vi "dfd_ZP Add Unit Circle and Axises.vi"(8 "error in (no error)":errorcluster, 10 "upper half plane only":bool, 11 "zero pole plot in":cluster{dbl[], dbl[]}[](array[cluster])) -> (0 "error out":errorcluster, 3 "zero pole plot out":cluster{dbl[], dbl[]}[](array[cluster]))   [LabVIEW 2017, in "NI_DigFilterLicensed.lvlib"]
uses:
  <vilib>/addons/Digital Filter Design/NI_DigFilterLicensed.lvlib
  <vilib>/Analysis/NI_AALBase.lvlib
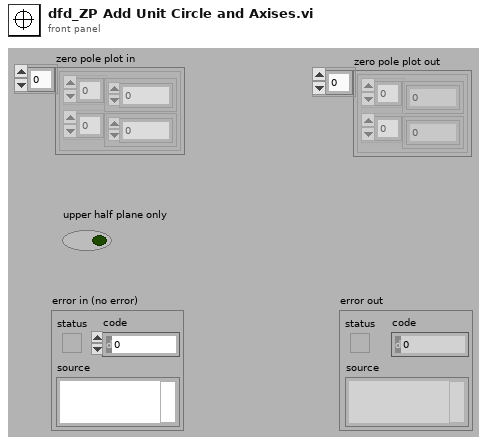
[diagram p1: front panel]
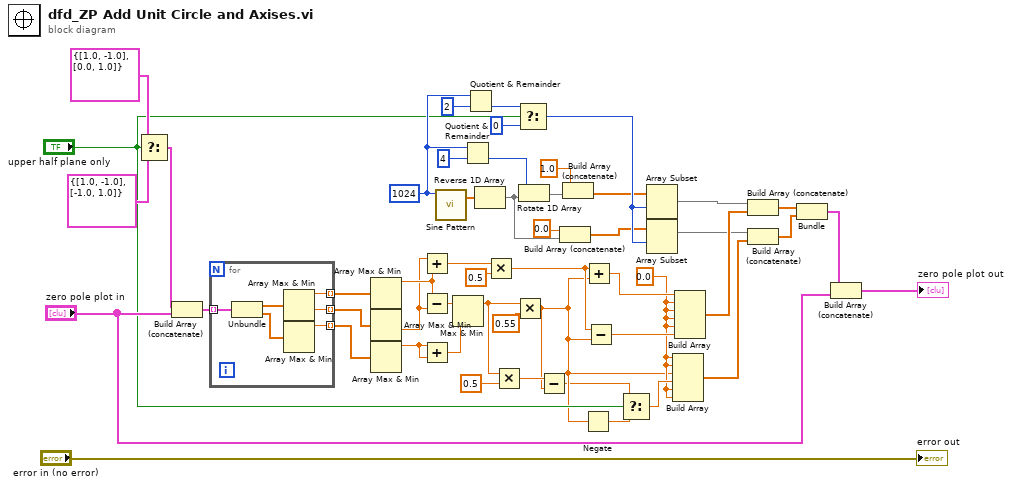
[diagram p0: block diagram]
diagram:
  w24 = 0.0 ("element")
  w22 = 1024 ("samples")
  n1 = Select(t=cluster{dbl[], dbl[]} {[1.0, -1.0], [0.0, 1.0]}, s="upper half plane only", f=cluster{dbl[], dbl[]} {[1.0, -1.0], [-1.0, 1.0]}) -> (s? t:f=w27:cluster{dbl[], dbl[]})
  n2 = Build Array (concatenate)(w27, "zero pole plot in") -> (w44:cluster{dbl[], dbl[]}[])
  n3 = for {
    tunnel: w44 -> [w57] mode=indexing
    tunnel: [w54] -> w42 mode=indexing
    tunnel: [w53] -> w41 mode=indexing
    tunnel: [w52] -> w40 mode=indexing
    n4 = Unbundle(w57) -> (w56:dbl[], w55:dbl[])
    n5 = Array Max & Min(array=w56) -> (max value=w54:dbl, min value=w53:dbl)  [unwired: 2 out]
    n6 = Array Max & Min(array=w55) -> (max value=w52:dbl)  [unwired: 3 out]
  }
  n7 = Array Max & Min(array=w42) -> (max value=w34:dbl)  [unwired: 3 out]
  n8 = Array Max & Min(array=w41) -> (min value=w33:dbl)  [unwired: 3 out]
  n9 = Array Max & Min(array=w40) -> (max value=w37:dbl)  [unwired: 3 out]
  n10 = Add(x=w33, y=w34) -> (x+y=w31:dbl)
  n11 = Subtract(x=w34, y=w33) -> (x-y=w39:dbl)
  n12 = Add(x=w37, y=w37) -> (x+y=w38:dbl)
  n13 = call <vilib>:"Sine Pattern.vi"("samples"=w22) -> ("Sinusoidal Pattern"=w10:dbl[])  [unwired: 3 in, 1 out]
  n14 = Max & Min(x=w39, y=w38) -> (max(x,y)=w19:dbl)  [unwired: 1 out]
  n15 = Quotient & Remainder(x=w22, y=4) -> (floor(x/y)=w9:i32)  [unwired: 1 out]
  n16 = Quotient & Remainder(x=w22, y=2) -> (floor(x/y)=w20:i32)  [unwired: 1 out]
  n17 = Reverse 1D Array(array=w10) -> (reversed array=w4:dbl[])
  n18 = Multiply(x=w31, y=0.5) -> (x*y=w30:dbl)
  n19 = Multiply(x=w19, y=0.5) -> (x*y=w17:dbl)
  n20 = Multiply(x=w19, y=0.55) -> (x*y=w16:dbl)
  n21 = Select(t=w20, s="upper half plane only", f=0) -> (s? t:f=w13:i32)
  n22 = Rotate 1D Array(1:w4, 2:w9) -> (0:w6:dbl[])
  n23 = Subtract(x=w17, y=w16) -> (x-y=w15:dbl)
  n24 = Build Array (concatenate)(0.0, w4) -> (w7:dbl[])
  n25 = Build Array (concatenate)(1.0, w6) -> (w5:dbl[])
  n26 = Negate(x=w16) -> (-x=w26:dbl)
  n27 = Add(x=w30, y=w16) -> (x+y=w49:dbl)
  n28 = Subtract(x=w30, y=w16) -> (x-y=w36:dbl)
  n29 = Select(t=w15, s="upper half plane only", f=w26) -> (s? t:f=w25:dbl)
  n30 = Array Subset(array=w5, index=w13) -> (w12:dbl[])  [unwired: 1 in]
  n31 = Array Subset(array=w7, index=w13) -> (w8:dbl[])  [unwired: 1 in]
  n32 = Build Array(w24, w24, w16, w25, w24, w24) -> (w11:dbl[])
  n33 = Build Array(w49, w24, w24, w24, w24, w36) -> (w48:dbl[])
  n34 = Build Array (concatenate)(w12, w48) -> (w47:dbl[])
  n35 = Build Array (concatenate)(w8, w11) -> (w46:dbl[])
  n36 = Bundle(w47, w46) -> (w1:cluster{dbl[], dbl[]})  [unwired: 1 out]
  n37 = Build Array (concatenate)(w1, "zero pole plot in") -> (→"zero pole plot out":cluster{dbl[], dbl[]}[])
  "error out" <- "error in (no error)"
